vi "Dialog Box - Resize Window.vi"(8 "error in (no error)":errorcluster, 9 "Height":i16, 10 "Width":i16, 11 "reference":refnum<vi>) -> (0 "error out":errorcluster)   [LabVIEW 2011]
doc: "Sets the size of a visible front panel. Also resets the default pane origin to 0,0."
uses:
  <vilib>/Utility/miscctls.llb/LVPointTypeDef.ctl
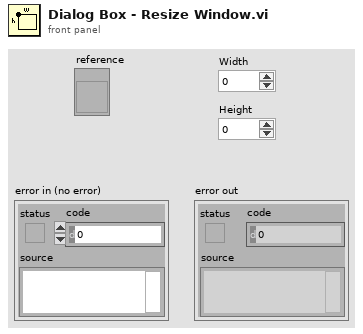
[diagram p1: front panel]
types:
  T1 = typedef "LVPointTypeDef.ctl" = cluster{"Horizontal":i16, "Vertical":i16}
  T2 = typedef "LVRectTypeDef.ctl" = cluster{"Left":i16, "Top":i16, "Right":i16, "Bottom":i16}
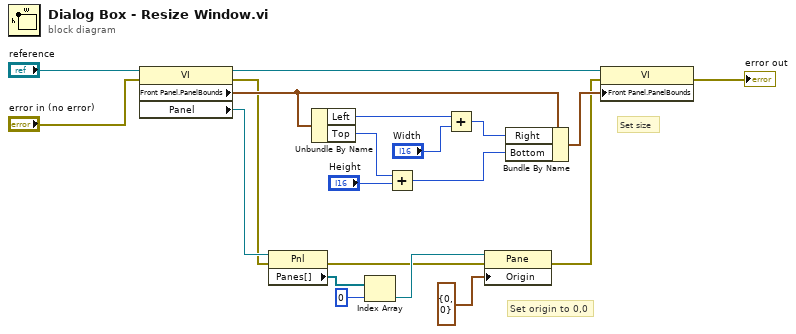
[diagram p0: block diagram]
diagram:
  # "Set origin to 0,0"
  # "Set size"
  n1 = property class="VI"(reference="reference", error in="error in (no error)") -> (reference out=w7:refnum<vi>, error out=w3:errorcluster, "Front Panel.PanelBounds"=w15:T2, "Panel"=w16:refnum<vi>)
  n2 = property class="Pnl"(reference=w16, error in=w3) -> (error out=w4:errorcluster, "Panes[]"=w17:refnum<vi>[])  [unwired: 1 out]
  n3 = Unbundle By Name(w15) -> ("Left"=w14:i16, "Top"=w10:i16)
  n4 = Index Array(array=w17, index=0) -> (element=w19:refnum<vi>)
  n5 = Add(x=w10, y="Height") -> (x+y=w11:i16)
  n6 = Add(x=w14, y="Width") -> (x+y=w13:i16)
  n7 = property class="Pane"(reference=w19, error in=w4, "Origin"=T1 {"Horizontal"=0, "Vertical"=0}) -> (error out=w2:errorcluster)  [unwired: 1 out]
  n8 = Bundle By Name(cluster=w15, "Right"=w13, "Bottom"=w11) -> (w6:T2)
  n9 = property class="VI"(reference=w7, error in=w2, "Front Panel.PanelBounds"=w6) -> (error out=→"error out":errorcluster)  [unwired: 1 out]
